vi "measure_digital_FPGA.vi"() -> ()   [LabVIEW 2018]
uses:
  <vilib>/rvi/Emulation/niFpgaGetClockAttributes.vi
  <vilib>/rvi/Emulation/niFpgaSctlEmulationGetInTimedLoop.vi
  <vilib>/rvi/Emulation/niFpgaEmulationReportErrorSimple.vi
  <vilib>/rvi/eio/common/nirviEmuTemplateMethod_errors.vi
  <vilib>/rvi/Emulation/niFpgaCriticalErrorInLSC.vi
  <vilib>/eio/EIONode/EIONode.xnode
panel:
  in  "Sampling Interval for  1MHz\nFrequency (us)":u32=1
  out "Period":u32
  # "Measure Period at \nConnector A/DIO1"
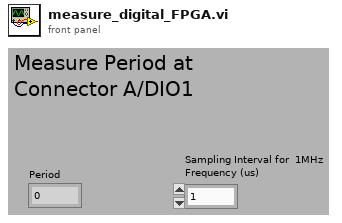
[diagram p1: front panel]
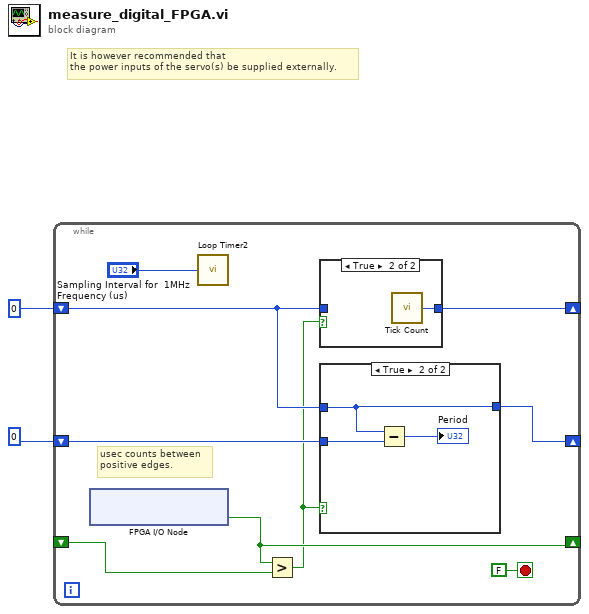
[diagram p0: block diagram]
diagram:
  # "It is however recommended that\nthe power inputs of the servo(s) be supplied externally."
  n1 = while {
    shift-right: [w6] -> _
    shift-left: _ -> [w11]
    shift-right: [w10] -> _
    shift-left: u32 0 ("Tick Count(Ticks)") -> [w5]
    shift-right: [w8] -> _
    shift-left: u32 0 ("Tick Count(Ticks)") -> [w9]
    stop <- FALSE stop-if-true
    # "usec counts between\npositive edges."
    n2 = xnode "FPGA I/O Node"() -> ("ConnectorA/DIO1"=w6:bool)  [unwired: 1 in, 1 out]
    n3 = call "Loop Timer2"("Count(uSec)"="Sampling Interval for  1MHz\nFrequency (us)") -> ()  [unwired: 1 out]
    n4 = Greater?(x=w6, y=w11) -> (0:w3:bool)
    n5 = case shown="True" w3 {
      tunnel: [w16 w17] -> w10
      tunnel: w5 -> [w16 _]
      frame False {
      }
      frame True {
        n6 = call "Tick Count"() -> ("Tick Count(uSec)"=w17:u32)
      }
    }
    n7 = case shown="True" w3 {
      tunnel: w9 -> [w12 w15]
      tunnel: [w12 w14] -> w8
      tunnel: w5 -> [_ w14]
      frame False {
      }
      frame True {
        n8 = Subtract(x=w14, y=w15) -> (x-y=→"Period":u32)
      }
    }
  }
